vi "Has Role.vi"(8 "error in (no error)":errorcluster, 9 "Description (None)":string, 10 "Role":string, 11 "Security in":refnum<class "Security.lvclass">) -> (0 "error out":errorcluster, 3 "Security out":refnum<class "Security.lvclass">)   [LabVIEW 2020, in "HTTP Server.lvlib" / "Security.lvclass"]
uses:
  Security.lvclass
  Security.lvclass/Security.ctl
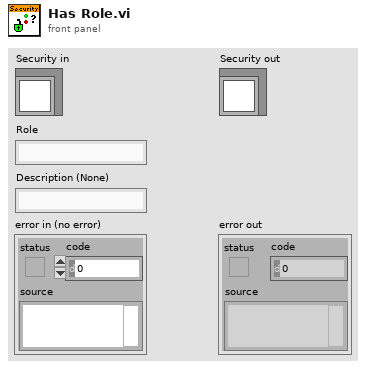
[diagram p1: front panel]
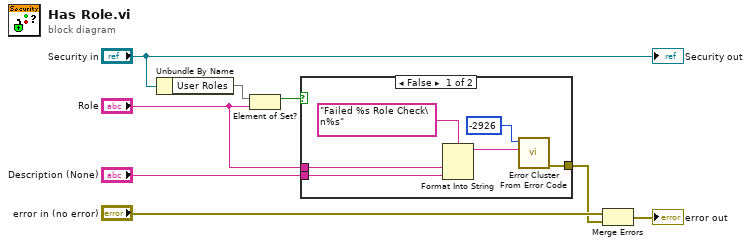
[diagram p0: block diagram]
diagram:
  n1 = Unbundle By Name("Security in") -> ("User Roles"=w6:set{string})
  n2 = Element of Set?(10:"Role", 11:w6) -> (3:w5:bool)
  n3 = case shown="False" w5 {
    tunnel: [w13 _] -> w3
    tunnel: "Role" -> [w11 _]
    tunnel: "Description (None)" -> [w10 _]
    frame False {
      n4 = Format Into String(format string="Failed %s Role Check\n%s", w11, w10) -> (resulting string=w9:string)  [unwired: 2 in, 1 out]
      n5 = call <vilib>:"Error Cluster From Error Code.vi"("error message (\"\")"=w9, "error code (0)"=-2926) -> ("error out"=w13:errorcluster)  [unwired: 7 in]
    }
    frame True {
    }
  }
  n6 = Merge Errors("error in (no error)", w3) -> (→"error out":errorcluster)
  "Security out" <- "Security in"
